vi "variant2Attributes.vi"(0 "HGF_PVDataConverter":refnum<class "HGF_PVDataConverter.lvclass">, 2 "rawData":variant, 3 "typeDescriptor":string, 5 "error in (no error)":errorcluster) -> (14 "HGF_PVDataConverter":refnum<class "HGF_PVDataConverter.lvclass">, 15 "no link":bool, 16 "Parameter":variant, 17 "typeDescriptor":string, 19 "error out":errorcluster)   [LabVIEW 2014, in "HGF_BaseClasses.lvlib" / "HGF_PVDataConverter.lvclass"]
doc: "Convert raw data value of variant to variant attributes Pn, n=0,1,2,..."
uses:
  HGF_PVDataConverter.lvclass
  HGF_Auxiliary/ErrorCode.ctl
  HGF_Auxiliary/Severity.ctl
  HGF_Auxiliary/HGF_Auxiliary.lvlib
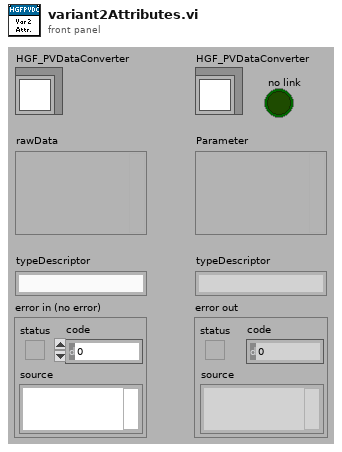
[diagram p1: front panel]
types:
  T1 = typedef "HGF_Auxiliary.lvlib/Severity.ctl" = enum16{"Info", "Warning", "Fault", "Error", "Fatal"}
  T2 = typedef "HGF_Auxiliary.lvlib/ErrorCode.ctl" = enum32{"No error", "Function not supported.", "This VI is for friends only.", "Reference object aready exisits.", "Parameter out of range.", "Not a rendezvous.", "Invalid notifier reference.", "Invalid queue reference.", "Self-Test not supported.", "Reset not supported.", "IDN query not supported.", "Error query not supported.", "Incorrect addressee.", "Object already exists.", "No class name specified", "Driver not supported", "Attribute is not writable"}
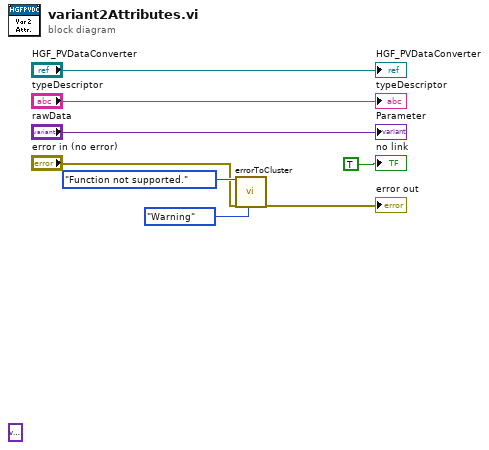
[diagram p0: block diagram]
diagram:
  (unwired) variant ("rawData")
  (unwired) variant ("rawData")
  n1 = call "errorToCluster.vi"("error code"=ErrorCode."Function not supported.", "error in (no error)"="error in (no error)", "severity (Error)"=Severity."Warning") -> ("error out"=→"error out":errorcluster)  [unwired: 2 in, 14 out]
  "HGF_PVDataConverter" <- "HGF_PVDataConverter"
  "Parameter" <- "rawData"
  "typeDescriptor" <- "typeDescriptor"
  "no link" <- TRUE ("no link")
